vi "LS Durability Main ORIGINAL (FPGA).vi"() -> ()   [LabVIEW 2013]
uses:
  <vilib>/rvi/Emulation/niFpgaSctlEmulationGetInTimedLoop.vi
  <vilib>/rvi/Emulation/niFpgaEmulationReportErrorSimple.vi
  <vilib>/rvi/Emulation/niFpgaGetClockAttributes.vi
  <vilib>/rvi/eio/common/nirviEmuTemplateMethod_errors.vi
  <vilib>/rvi/Emulation/niFpgaCriticalErrorInLSC.vi
  <vilib>/eio/EIONode/EIONode.xnode
panel:
  out "AI Loop Time (usec)":u32=70
  out "Analog Inputs":fxp<+/-,28,17>[](array[numeric])
  in  "Enable Readings":bool[](array[boolean])=[FALSE, FALSE, FALSE, FALSE, FALSE, FALSE, FALSE, FALSE, FALSE, FALSE, FALSE, FALSE]
  in  "PWM Period (Ticks)":u32=4000000
  in  "Duty (Ticks)":i32=2000000
  in  "Invert PWM?":bool=TRUE
  in  "Bank1(Pulse/Const)":bool
  in  "Bank1Const(On/Off)":bool
  in  "Bank2(Pulse/Const)":bool
  in  "Bank2Const(On/Off)":bool
  out "Bank1On":bool
  out "Bank2On":bool
  out "Opens Loop Time (usec)":u32=1000
  out "Opens Detected":i16[](array[numeric])
  in  "Enable Opens":bool[](array[boolean])=[FALSE, FALSE, FALSE, FALSE, FALSE, FALSE, FALSE, FALSE, FALSE, FALSE, FALSE, FALSE]
  in  "Opens Resets":bool[](array[boolean])=[FALSE, FALSE, FALSE, FALSE, FALSE, FALSE, FALSE, FALSE, FALSE, FALSE, FALSE, FALSE]
  out "Anomalies (Last Cycle)":i32[](array[numeric])=[12, 0, 0, 0, 0, 0, 0, 0, 0, 0, 0, 0]
  out "Cycle Starts":bool[](array[boolean])
  out "Anomalies (Total)":i32[](array[numeric])=[12, 0, 0, 0, 0, 0, 0, 0, 0, 0, 0, 0]
  out "Anomalies/Cycle":i32[](array[numeric])=[12, 0, 0, 0, 0, 0, 0, 0, 0, 0, 0, 0]
  in  "Normal Steps":u32=98
  out "Cycles":u32[](array[numeric])=[12, 0, 0, 0, 0, 0, 0, 0, 0, 0, 0, 0]
  out "Anomaly Loop Time (usec)":u32=1000
  out "Steps":u32[](array[numeric])=[117, 0, 0, 0, 0, 0, 0, 0, 0, 0, 0, 0]
  in  "Anomaly Threshold":fxp<+/-,28,17>=0.02978515625
  in  "Enable Anomalies":bool[](array[boolean])=[TRUE, FALSE, FALSE, FALSE, FALSE, FALSE, FALSE, FALSE, FALSE, FALSE, FALSE, FALSE]
  in  "Anomaly Resets":bool[](array[boolean])=[FALSE, FALSE, FALSE, FALSE, FALSE, FALSE, FALSE, FALSE, FALSE, FALSE, FALSE, FALSE]
  in  "Cycle Resets":bool[](array[boolean])=[FALSE, FALSE, FALSE, FALSE, FALSE, FALSE, FALSE, FALSE, FALSE, FALSE, FALSE, FALSE]
  in  "Points to Avg":i32=20
  in  "Enable Cycles":bool[](array[boolean])=[TRUE, FALSE, FALSE, FALSE, FALSE, FALSE, FALSE, FALSE, FALSE, FALSE, FALSE, FALSE]
  out "Total Cycles":u32[](array[numeric])=[12, 0, 0, 0, 0, 0, 0, 0, 0, 0, 0, 0]
  in  "Cycle Threshold":fxp<+/-,28,17>=1.2001953125
  out "AI Avg Loop Time (usec)":u32=1000
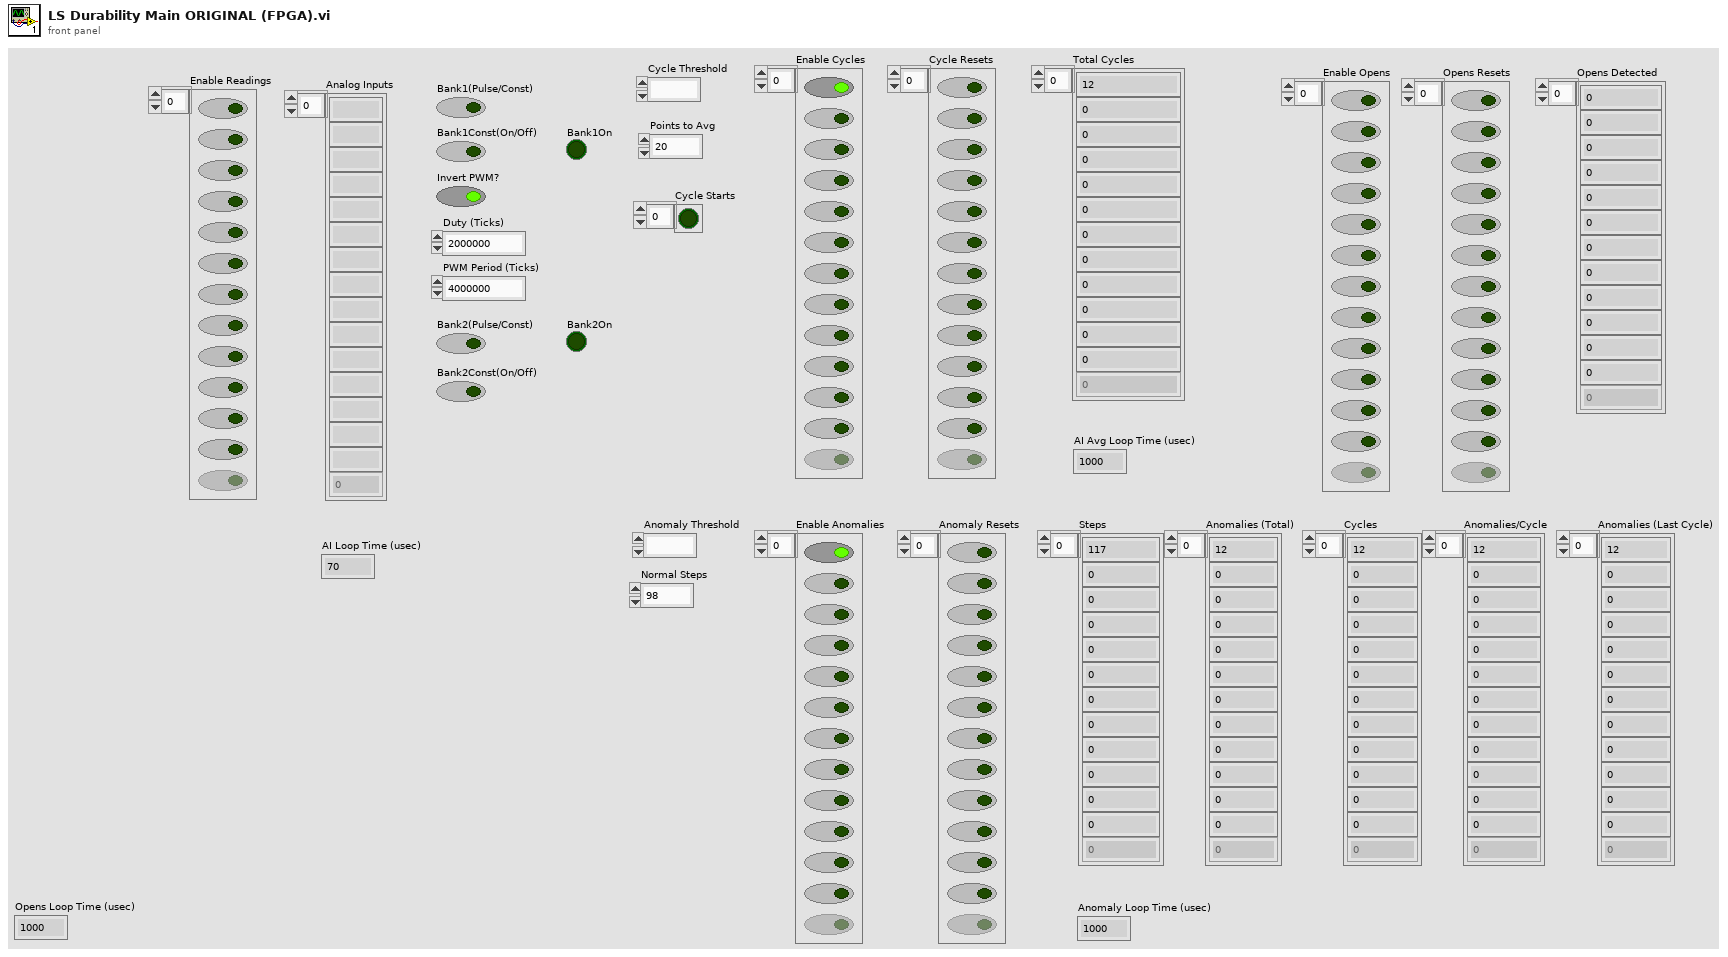
[diagram p1: front panel]
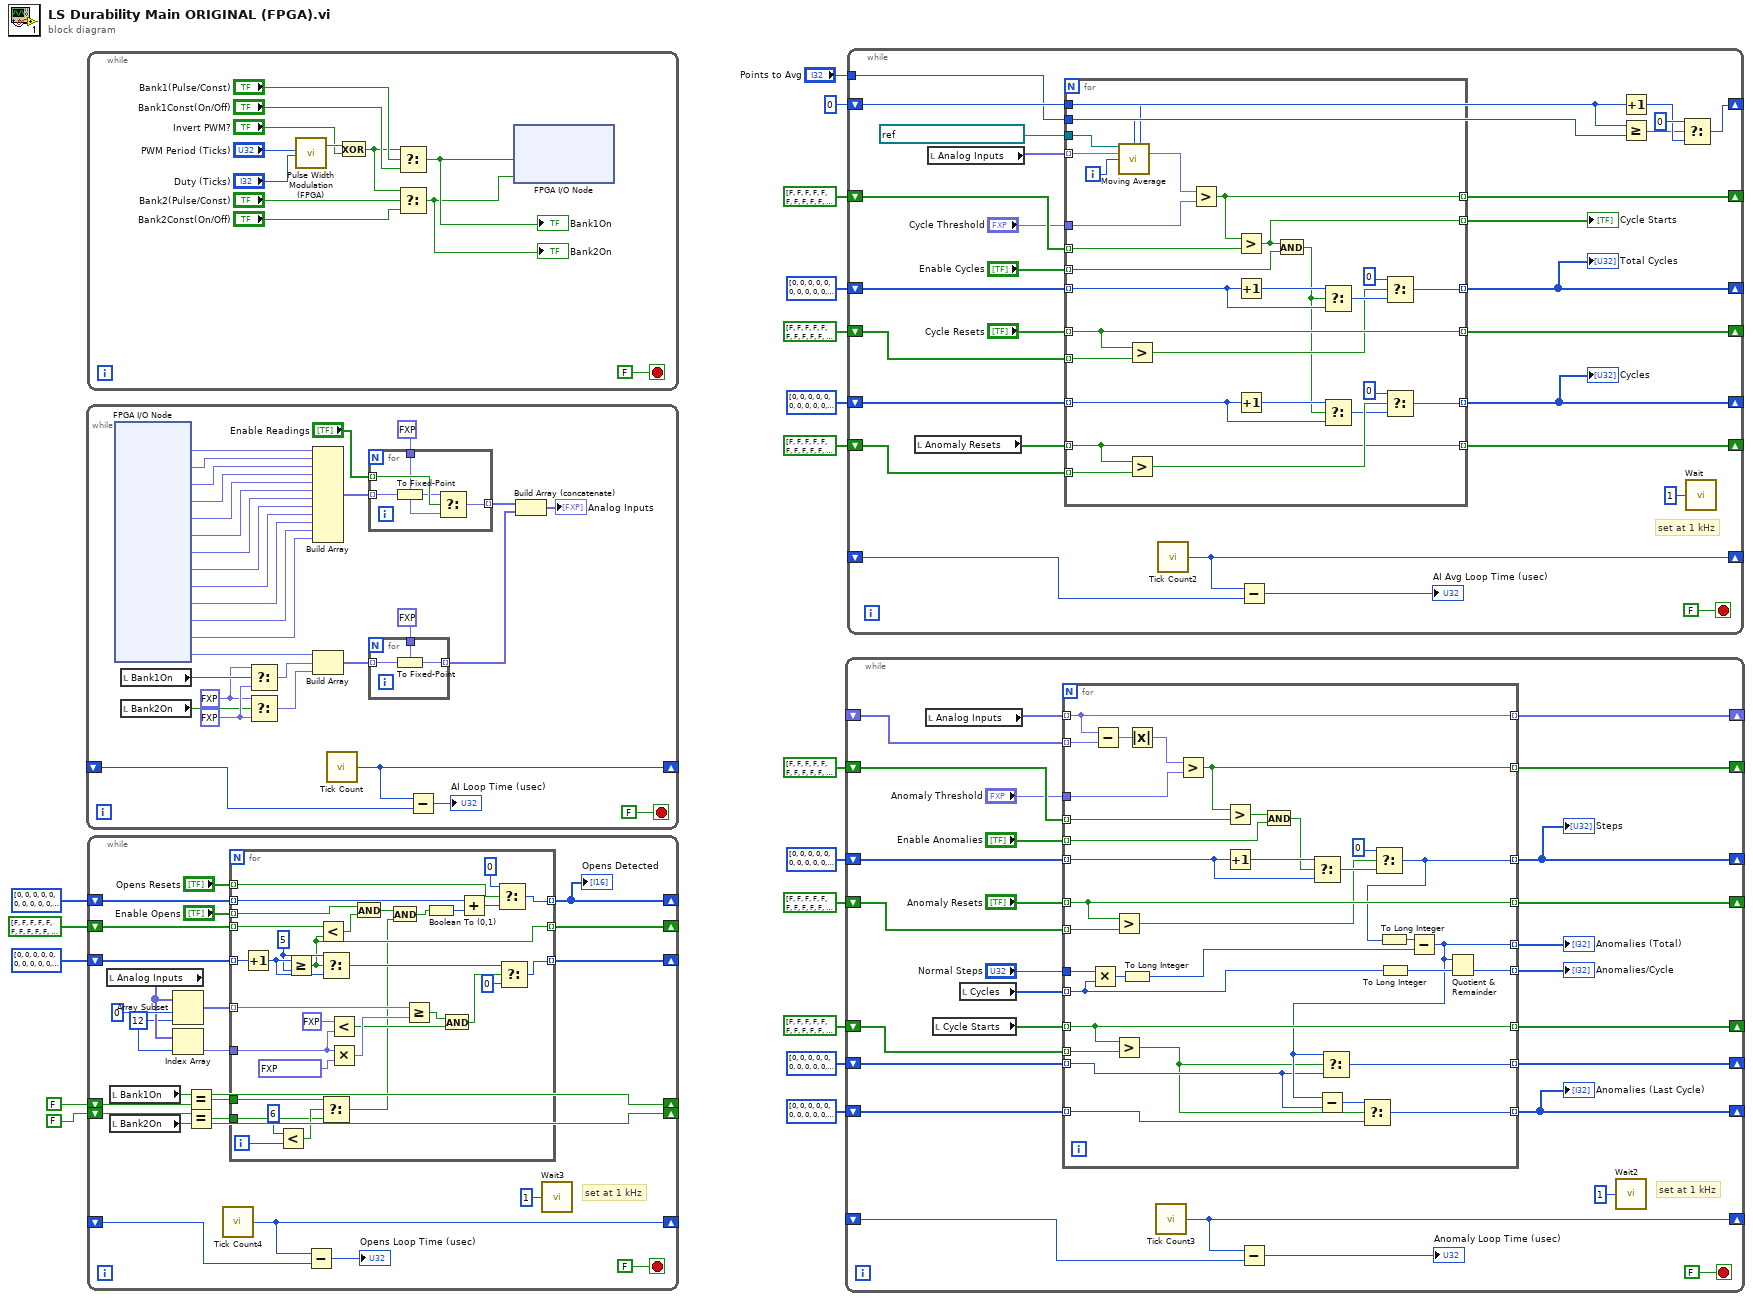
[diagram p0: block diagram]
diagram:
  n1 = while {
    shift-right: [w48] -> _
    shift-left: _ -> [w47]
    stop <- FALSE stop-if-true
    w21 = fxp<+/-,24,5> 1.0 ("AI13")
    w24 = fxp<+/-,24,5> 0.0 ("AI13")
    n2 = xnode "FPGA I/O Node"() -> ("AI0"=w45:fxp<+/-,24,5>, "AI1"=w44:fxp<+/-,24,5>, "AI2"=w43:fxp<+/-,24,5>, "AI3"=w42:fxp<+/-,24,5>, "AI4"=w41:fxp<+/-,24,5>, "AI5"=w40:fxp<+/-,24,5>, "AI6"=w39:fxp<+/-,24,5>, "AI7"=w38:fxp<+/-,24,5>, "AI8"=w37:fxp<+/-,24,5>, "AI9"=w36:fxp<+/-,24,5>, "AI10"=w35:fxp<+/-,24,5>, "AI11"=w34:fxp<+/-,24,5>, "AI12"=w31:fxp<+/-,24,5>)  [unwired: 13 in, 13 out]
    n3 = local read "Bank1On"() -> (w23:bool)
    n4 = local read "Bank2On"() -> (w22:bool)
    n5 = Select(t=w21, s=w23, f=w24) -> (s? t:f=w20:fxp<+/-,24,5>)
    n6 = Select(t=w21, s=w22, f=w24) -> (s? t:f=w19:fxp<+/-,24,5>)
    n7 = Build Array(w45, w44, w43, w42, w41, w40, w39, w38, w37, w36, w35, w34) -> (w33:fxp<+/-,24,5>[])
    n8 = Build Array(w31, w20, w19) -> (w29:fxp<+/-,24,5>[])
    n9 = call "Tick Count"() -> ("Tick Count(uSec)"=w48:u32)
    n10 = for {
      tunnel: w33 -> [w57] mode=indexing
      tunnel: fxp<+/-,28,17> 0.0 ("AI0") -> [w54]
      tunnel: [w53] -> w27 mode=indexing
      tunnel: "Enable Readings" -> [w56] mode=indexing
      n11 = To Fixed-Point(fixed-point type=w54, number=w57) -> (fixed-point=w55:fxp<+/-,28,17>)
      n12 = Select(t=w55, s=w56, f=w54) -> (s? t:f=w53:fxp<+/-,28,17>)
    }
    n13 = for {
      tunnel: w29 -> [w52] mode=indexing
      tunnel: fxp<+/-,28,17> 0.0 ("AI0") -> [w51]
      tunnel: [w50] -> w28 mode=indexing
      n14 = To Fixed-Point(fixed-point type=w51, number=w52) -> (fixed-point=w50:fxp<+/-,28,17>)
    }
    n15 = Subtract(x=w48, y=w47) -> (x-y=→"AI Loop Time (usec)":u32)
    n16 = Build Array (concatenate)(w27, w28) -> (→"Analog Inputs":fxp<+/-,28,17>[])
  }
  n17 = while {
    stop <- FALSE stop-if-true
    n18 = call "Pulse Width Modulation (FPGA).vi"("PWM Period (Ticks)"="PWM Period (Ticks)", "PWM Duty Cycle (Ticks)"="Duty (Ticks)") -> ("PWM DO"=w66:bool)  [unwired: 14 in, 3 out]
    n19 = Exclusive Or(1:"Invert PWM?", 2:w66) -> (0:w62:bool)
    n20 = Select(t=w62, s="Bank1(Pulse/Const)", f="Bank1Const(On/Off)") -> (s? t:f=w59:bool)
    "Bank1On" <- w59
    n21 = Select(t=w62, s="Bank2(Pulse/Const)", f="Bank2Const(On/Off)") -> (s? t:f=w58:bool)
    "Bank2On" <- w58
    n22 = xnode "FPGA I/O Node"("RMC/DIO0"=w59, "RMC/DIO1"=w58) -> ()  [unwired: 3 in, 3 out]
  }
  n23 = while {
    shift-right: [w90] -> _
    shift-left: _ -> [w89]
    shift-right: [w84] -> _
    shift-left: bool[] [FALSE, FALSE, FALSE, FALSE, FALSE, FALSE, FALSE, FALSE, FALSE, FALSE, FALSE, FALSE] -> [w86]
    shift-right: [w80] -> _
    shift-left: i16[] [0, 0, 0, 0, 0, 0, 0, 0, 0, 0, 0, 0] -> [w83]
    shift-right: [w81] -> _
    shift-left: i16[] [0, 0, 0, 0, 0, 0, 0, 0, 0, 0, 0, 0] -> [w82]
    shift-right: [w72] -> _
    shift-left: FALSE -> [w75]
    shift-right: [w73] -> _
    shift-left: FALSE -> [w74]
    stop <- FALSE stop-if-true
    w76 = 12 ("length")
    # "set at 1 kHz"
    n24 = local read "Analog Inputs"() -> (w85:fxp<+/-,28,17>[])
    n25 = local read "Bank1On"() -> (w72:bool)
    n26 = local read "Bank2On"() -> (w73:bool)
    n27 = Array Subset(array=w85, index=0, length=w76) -> (w79:fxp<+/-,28,17>[])
    n28 = Index Array(array=w85, index=w76) -> (element=w87:fxp<+/-,28,17>)
    n29 = Equal?(x=w72, y=w75) -> (x = y?=w71:bool)
    n30 = Equal?(x=w74, y=w73) -> (x = y?=w70:bool)
    n31 = call "Tick Count4"() -> ("Tick Count(uSec)"=w90:u32)
    n32 = for {
      tunnel: w79 -> [w106] mode=indexing
      tunnel: w87 -> [w102]
      tunnel: w86 -> [w125] mode=indexing
      tunnel: [w110] -> w84 mode=indexing
      tunnel: w83 -> [w121] mode=indexing
      tunnel: [w108] -> w80 mode=indexing
      tunnel: "Enable Opens" -> [w119] mode=indexing
      tunnel: "Opens Resets" -> [w117] mode=indexing
      tunnel: w82 -> [w114] mode=indexing
      tunnel: [w109] -> w81 mode=indexing
      tunnel: w71 -> [w100]
      tunnel: w70 -> [w99]
      i -> [w97]
      w111 = i16 5 ("y")
      n33 = Increment(x=w114) -> (x+1=w112:i16)
      n34 = Less?(x=6 ("y"), y=w97) -> (x < y?=w101:bool)
      n35 = Greater Or Equal?(x=w112, y=w111) -> (x >= y?=w110:bool)
      n36 = Less?(x=w125, y=w110) -> (x < y?=w120:bool)
      n37 = Select(t=w111, s=w110, f=w112) -> (s? t:f=w113:i16)
      n38 = Select(t=w100, s=w101, f=w99) -> (s? t:f=w94:bool)
      n39 = Less?(x=fxp<+/-,28,17> 1.0, y=w102) -> (x < y?=w103:bool)
      n40 = Multiply(x=w102, y=fxp<+,8,0> 0.94921875) -> (x*y=w123:fxp<+/-,36,17>)
      n41 = And(x=w119, y=w120) -> (x .and. y?=w96:bool)
      n42 = And(x=w96, y=w94) -> (x .and. y?=w95:bool)
      n43 = Greater Or Equal?(x=w106, y=w123) -> (x >= y?=w104:bool)
      n44 = Boolean To (0,1)(Boolean=w95) -> (0, 1=w122:i16)
      n45 = And(x=w104, y=w103) -> (x .and. y?=w107:bool)
      n46 = Add(x=w121, y=w122) -> (x+y=w118:i16)
      n47 = Select(t=i16 0, s=w117, f=w118) -> (s? t:f=w108:i16)
      n48 = Select(t=w113, s=w107, f=i16 0) -> (s? t:f=w109:i16)
    }
    "Opens Detected" <- w80
    n49 = Subtract(x=w90, y=w89) -> (x-y=→"Opens Loop Time (usec)":u32)
    n50 = call "Wait3"("Count(mSec)"=u32 1) -> ()  [unwired: 1 out]
  }
  n51 = while {
    shift-right: [w149] -> _
    shift-left: _ -> [w148]
    shift-right: [w147] -> _
    shift-left: bool[] [FALSE, FALSE, FALSE, FALSE, FALSE, FALSE, FALSE, FALSE, FALSE, FALSE, FALSE, FALSE] -> [w146]
    shift-right: [w136] -> _
    shift-left: u32[] [0, 0, 0, 0, 0, 0, 0, 0, 0, 0, 0, 0] -> [w145]
    shift-right: [w141] -> _
    shift-left: bool[] [FALSE, FALSE, FALSE, FALSE, FALSE, FALSE, FALSE, FALSE, FALSE, FALSE, FALSE, FALSE] -> [w140]
    shift-right: [w139] -> _
    shift-left: _ -> [w138]
    shift-right: [w131] -> _
    shift-left: bool[] [FALSE, FALSE, FALSE, FALSE, FALSE, FALSE, FALSE, FALSE, FALSE, FALSE, FALSE, FALSE] -> [w130]
    shift-right: [w129] -> _
    shift-left: i32[] [0, 0, 0, 0, 0, 0, 0, 0, 0, 0, 0, 0] -> [w128]
    shift-right: [w126] -> _
    shift-left: i32[] [0, 0, 0, 0, 0, 0, 0, 0, 0, 0, 0, 0] -> [w127]
    stop <- FALSE stop-if-true
    # "set at 1 kHz"
    n52 = local read "Analog Inputs"() -> (w151:fxp<+/-,28,17>[])
    n53 = local read "Cycle Starts"() -> (w132:bool[])
    n54 = local read "Cycles"() -> (w135:u32[])
    n55 = for {
      tunnel: w151 -> [w174] mode=indexing
      tunnel: [w187] -> w147 mode=indexing
      tunnel: w146 -> [w186] mode=indexing
      tunnel: w145 -> [w170] mode=indexing
      tunnel: [w166] -> w136 mode=indexing
      tunnel: "Anomaly Threshold" -> [w184]
      tunnel: "Enable Anomalies" -> [w182] mode=indexing
      tunnel: "Anomaly Resets" -> [w180] mode=indexing
      tunnel: [w180] -> w141 mode=indexing
      tunnel: w140 -> [w179] mode=indexing
      tunnel: [w174] -> w139 mode=indexing
      tunnel: w138 -> [w173] mode=indexing
      tunnel: "Normal Steps" -> [w171]
      tunnel: w135 -> [w164] mode=indexing
      tunnel: [w163] -> w133 mode=indexing
      tunnel: [w159] -> w134 mode=indexing
      tunnel: w132 -> [w162] mode=indexing
      tunnel: [w162] -> w131 mode=indexing
      tunnel: w130 -> [w161] mode=indexing
      tunnel: [w160] -> w129 mode=indexing
      tunnel: w128 -> [w158] mode=indexing
      tunnel: [w155] -> w126 mode=indexing
      tunnel: w127 -> [w154] mode=indexing
      n56 = Multiply(x=w171, y=w164) -> (x*y=w169:u32)
      n57 = Subtract(x=w174, y=w173) -> (x-y=w175:fxp<+/-,29,18>)
      n58 = Greater?(x=w180, y=w179) -> (0:w177:bool)
      n59 = Greater?(x=w162, y=w161) -> (0:w156:bool)
      n60 = To Long Integer(number=w169) -> (32bit integer=w165:i32)
      n61 = Absolute Value(x=w175) -> (abs(x)=w172:fxp<+,28,17>)
      n62 = Greater?(x=w172, y=w184) -> (0:w187:bool)
      n63 = Greater?(x=w187, y=w186) -> (0:w183:bool)
      n64 = Increment(x=w170) -> (x+1=w185:u32)
      n65 = And(x=w183, y=w182) -> (x .and. y?=w181:bool)
      n66 = Select(t=w185, s=w181, f=w170) -> (s? t:f=w178:u32)
      n67 = Select(t=u32 0, s=w177, f=w178) -> (s? t:f=w166:u32)
      n68 = To Long Integer(number=w166) -> (32bit integer=w168:i32)
      n69 = To Long Integer(number=w164) -> (32bit integer=w167:i32)
      n70 = Subtract(x=w168, y=w165) -> (x-y=w159:i32)
      n71 = Subtract(x=w159, y=w158) -> (x-y=w157:i32)
      n72 = Select(t=w159, s=w156, f=w158) -> (s? t:f=w160:i32)
      n73 = Select(t=w157, s=w156, f=w154) -> (s? t:f=w155:i32)
      n74 = Quotient & Remainder(x=w159, y=w167) -> (floor(x/y)=w163:i32)  [unwired: 1 out]
    }
    "Steps" <- w136
    "Anomalies/Cycle" <- w133
    "Anomalies (Total)" <- w134
    "Anomalies (Last Cycle)" <- w126
    n75 = call "Tick Count3"() -> ("Tick Count(uSec)"=w149:u32)
    n76 = Subtract(x=w149, y=w148) -> (x-y=→"Anomaly Loop Time (usec)":u32)
    n77 = call "Wait2"("Count(mSec)"=u32 1) -> ()  [unwired: 1 out]
  }
  n78 = while {
    shift-right: [w209] -> _
    shift-left: 0 ("Moving Point Index") -> [w210]
    shift-right: [w205] -> _
    shift-left: _ -> [w204]
    shift-right: [w203] -> _
    shift-left: bool[] [FALSE, FALSE, FALSE, FALSE, FALSE, FALSE, FALSE, FALSE, FALSE, FALSE, FALSE, FALSE] -> [w202]
    shift-right: [w200] -> _
    shift-left: u32[] [0, 0, 0, 0, 0, 0, 0, 0, 0, 0, 0, 0] -> [w201]
    tunnel: "Points to Avg" -> [w197]
    shift-right: [w195] -> _
    shift-left: bool[] [FALSE, FALSE, FALSE, FALSE, FALSE, FALSE, FALSE, FALSE, FALSE, FALSE, FALSE, FALSE] -> [w194]
    shift-right: [w189] -> _
    shift-left: u32[] [0, 0, 0, 0, 0, 0, 0, 0, 0, 0, 0, 0] -> [w191]
    shift-right: [w192] -> _
    shift-left: bool[] [FALSE, FALSE, FALSE, FALSE, FALSE, FALSE, FALSE, FALSE, FALSE, FALSE, FALSE, FALSE] -> [w193]
    stop <- FALSE stop-if-true
    # "set at 1 kHz"
    n79 = local read "Anomaly Resets"() -> (w190:bool[])
    n80 = local read "Analog Inputs"() -> (w207:fxp<+/-,28,17>[])
    n81 = for {
      tunnel: w210 -> [w239]
      tunnel: w197 -> [w240]
      tunnel: w207 -> [w243] mode=indexing
      tunnel: refnum<k21> "Running Avg Memory" ("Memory") -> [w242]
      tunnel: [w237] -> w203 mode=indexing
      tunnel: w202 -> [w236] mode=indexing
      tunnel: w201 -> [w234] mode=indexing
      tunnel: [w226] -> w200 mode=indexing
      tunnel: "Cycle Threshold" -> [w233]
      tunnel: "Enable Cycles" -> [w232] mode=indexing
      tunnel: "Cycle Resets" -> [w231] mode=indexing
      tunnel: [w231] -> w195 mode=indexing
      tunnel: w194 -> [w230] mode=indexing
      tunnel: w191 -> [w219] mode=indexing
      tunnel: [w225] -> w189 mode=indexing
      tunnel: w190 -> [w220] mode=indexing
      tunnel: [w220] -> w192 mode=indexing
      tunnel: w193 -> [w221] mode=indexing
      tunnel: [w216] -> w188 mode=indexing
      i -> [w241]
      n82 = call "Moving Average.vi"("Memory In"=w242, "N (# of Ave Pts 127 max)"=w240, "Moving Point Index"=w239, "Data IN"=w243, "Channel#"=w241) -> ("Averaged Data"=w238:fxp<+/-,28,17>)  [unwired: 10 in]
      n83 = Greater?(x=w231, y=w230) -> (0:w228:bool)
      n84 = Greater?(x=w220, y=w221) -> (0:w223:bool)
      n85 = Greater?(x=w238, y=w233) -> (0:w237:bool)
      n86 = Greater?(x=w237, y=w236) -> (0:w216:bool)
      n87 = Increment(x=w234) -> (x+1=w235:u32)
      n88 = Increment(x=w219) -> (x+1=w218:u32)
      n89 = And(x=w216, y=w232) -> (x .and. y?=w217:bool)
      n90 = Select(t=w235, s=w217, f=w234) -> (s? t:f=w229:u32)
      n91 = Select(t=w218, s=w217, f=w219) -> (s? t:f=w222:u32)
      n92 = Select(t=u32 0, s=w228, f=w229) -> (s? t:f=w226:u32)
      n93 = Select(t=u32 0, s=w223, f=w222) -> (s? t:f=w225:u32)
    }
    "Total Cycles" <- w200
    "Cycles" <- w189
    "Cycle Starts" <- w188
    n94 = call "Tick Count2"() -> ("Tick Count(uSec)"=w205:u32)
    n95 = Subtract(x=w205, y=w204) -> (x-y=→"AI Avg Loop Time (usec)":u32)
    n96 = Increment(x=w210) -> (x+1=w212:i32)
    n97 = Greater Or Equal?(x=w210, y=w197) -> (x >= y?=w211:bool)
    n98 = Select(t=0, s=w211, f=w212) -> (s? t:f=w209:i32)
    n99 = call "Wait"("Count(mSec)"=u32 1) -> ()  [unwired: 1 out]
  }
